vi "calibrateSignalsTest.vi"(7 "Analizator?":bool, 8 "ErrorIn":errorcluster, 11 "AccelerationDataIn":waveform(dbl)[](array[waveform])) -> (0 "ErrorOut":errorcluster, 3 "AccelerationDataOut":waveform(dbl)[](array[waveform]))   [LabVIEW 2019]
uses:
  <vilib>/Analysis/baseanly.llb/Mean (DBL).vi
  <vilib>/Analysis/NI_AALBase.lvlib
panel:
  in  "Czułość karta / analizator [V/g]":dbl[][](array[numeric])=[[0.1, 0.206], [0.1, 0.206], [0.1, 0.206]]
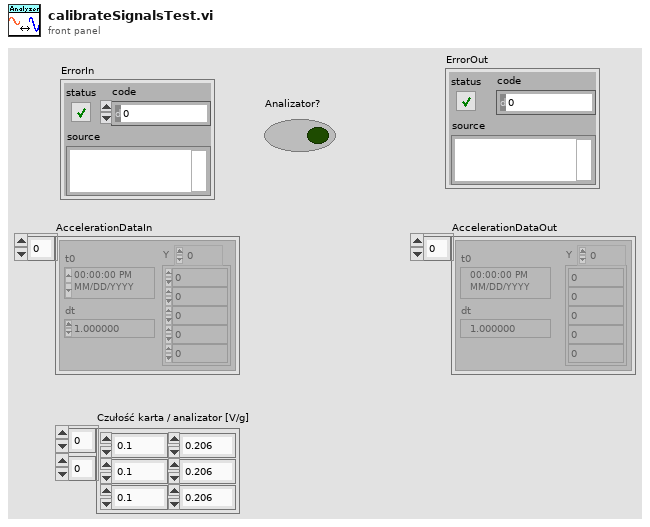
[diagram p1: front panel]
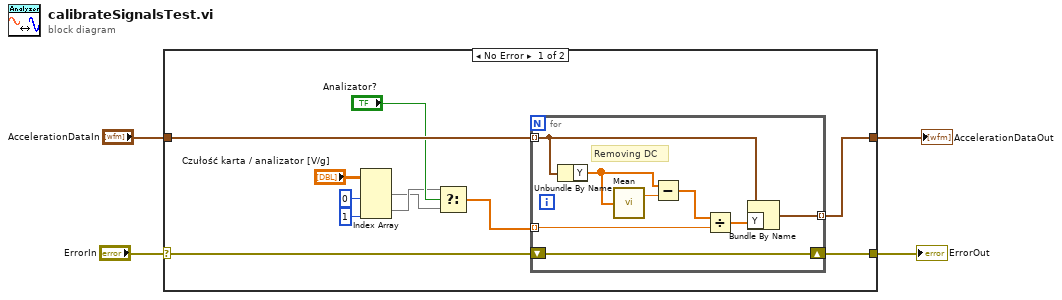
[diagram p0: block diagram]
diagram:
  n1 = case shown="No Error" "ErrorIn" {
    selector: "ErrorIn" -> [w15 w25]
    tunnel: "AccelerationDataIn" -> [w14 w24]
    tunnel: [w13 w25] -> w4
    tunnel: [w12 w24] -> w1
    frame No Error {
      n2 = Index Array(array="Czułość karta / analizator [V/g]", index (col) #1=0 ("disabled index (col)"), index (col) #2=1 ("index (col)")) -> (element #1=w6:dbl[], element #2=w7:dbl[])  [unwired: 2 in]
      n3 = Select(t=w7, s="Analizator?", f=w6) -> (s? t:f=w5:dbl[])
      n4 = for {
        tunnel: w14 -> [w17] mode=indexing
        shift-right: [w23] -> w13
        shift-left: w15 -> [w23]
        tunnel: w5 -> [w20] mode=indexing
        tunnel: [w16] -> w12 mode=indexing
        # "Removing DC"
        n5 = Unbundle By Name(w17) -> ("Y"=w22:dbl[])
        n6 = call-poly <vilib>:"Mean.vi"("X"=w22) -> ("mean"=w21:dbl)  [unwired: 1 out]
        n7 = Subtract(x=w22, y=w21) -> (x-y=w19:dbl[])
        n8 = Divide(x=w19, y=w20) -> (x/y=w18:dbl[])
        n9 = Bundle By Name(cluster=w17, "Y"=w18) -> (w16:waveform(dbl))
      }
    }
    frame Error {
    }
  }
  "ErrorOut" <- w4
  "AccelerationDataOut" <- w1
